vi "Rohde & Schwarz VNA Set Trace Display.vi"(4 "Trace":i8=1 min=1 max=99 step=1, 6 "Channel":i8=1 min=1 max=99 step=1, 7 "Rohde & Schwarz VNA":T1, 8 "error in (no error)":errorcluster, 11 "VISA Resource Name":refnum<visa-resource-name>) -> (0 "error out":errorcluster, 3 "dup VISA Resource Name":refnum<visa-resource-name>)   [LabVIEW 2011]
uses:
  TypeDefs/Rohde & Schwarz VNA Instrument Info.ctl
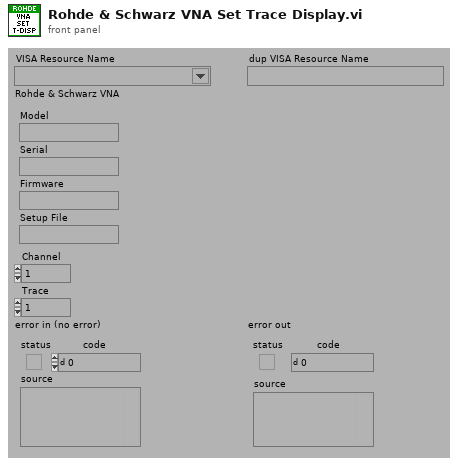
[diagram p1: front panel]
types:
  T1 = typedef "Rohde & Schwarz VNA Instrument Info.ctl" = cluster{"Model":string, "Serial":string, "Firmware":string, "Setup File":string}
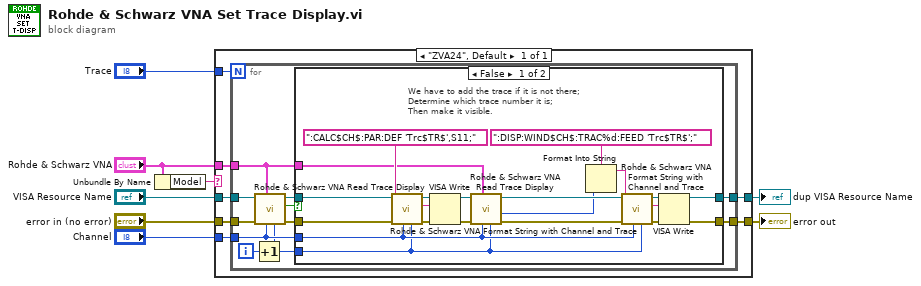
[diagram p0: block diagram]
diagram:
  n1 = Unbundle By Name("Rohde & Schwarz VNA") -> ("Model"=w1:string)
  n2 = case shown="\"ZVA24\", Default" w1 {
    tunnel: "VISA Resource Name" -> [w12]
    tunnel: "error in (no error)" -> [w13]
    tunnel: [w15] -> w6
    tunnel: [w14] -> w5
    tunnel: "Channel" -> [w10]
    tunnel: "Rohde & Schwarz VNA" -> [w11]
    tunnel: "Trace" -> [w9]
    frame "ZVA24", Default {
      n3 = for {
        N: w9 -> [_]
        tunnel: [w26] -> w15
        tunnel: [w25] -> w14
        tunnel: w13 -> [w24]
        tunnel: w12 -> [w23]
        tunnel: w11 -> [w18]
        tunnel: w10 -> [w17]
        i -> [w19]
        n4 = Increment(x=w19) -> (x+1=w16:i32)
        n5 = call "Rohde & Schwarz VNA Read Trace Display.vi"("Trace"=w16, "Channel"=w17, "Rohde & Schwarz VNA"=w18, "error in (no error)"=w24, "VISA Resource Name"=w23) -> ("error out"=w21:errorcluster, "Displayed?"=w20:bool, "dup VISA Resource Name"=w22:refnum<visa-resource-name>)  [unwired: 4 out]
        n6 = case shown="False" w20 {
          tunnel: [w36 w45] -> w26
          tunnel: [w35 w44] -> w25
          tunnel: w22 -> [w43 w45]
          tunnel: w21 -> [w42 w44]
          tunnel: w18 -> [w30 _]
          tunnel: w17 -> [w28 _]
          tunnel: w16 -> [w27 _]
          frame False {
            # "We have to add the trace if it is not there;\nDetermine which trace number it is;\nThen make it visible."
            n7 = call "Rohde & Schwarz VNA Format String with Channel and Trace.vi"("Trace"=w27, "Channel"=w28, "String"=":CALC$CH$:PAR:DEF 'Trc$TR$',S11;" ("write buffer")) -> ("String Out"=w41:string)  [unwired: 6 out]
            n8 = VISA Write(VISA resource name=w43, write buffer=w41, error in (no error)=w42) -> (VISA resource name out=w34:refnum<visa-resource-name>, error out=w33:errorcluster)  [unwired: 1 out]
            n9 = call "Rohde & Schwarz VNA Read Trace Display.vi"("Trace"=w27, "Channel"=w28, "Rohde & Schwarz VNA"=w30, "error in (no error)"=w33, "VISA Resource Name"=w34) -> ("error out"=w32:errorcluster, "Trace Index"=w29:i32, "dup VISA Resource Name"=w31:refnum<visa-resource-name>)  [unwired: 4 out]
            n10 = Format Into String(format string=":DISP:WIND$CH$:TRAC%d:FEED 'Trc$TR$';" ("write buffer"), w29) -> (resulting string=w38:string)  [unwired: 2 in, 1 out]
            n11 = call "Rohde & Schwarz VNA Format String with Channel and Trace.vi"("Trace"=w27, "Channel"=w28, "String"=w38) -> ("String Out"=w37:string)  [unwired: 6 out]
            n12 = VISA Write(VISA resource name=w31, write buffer=w37, error in (no error)=w32) -> (VISA resource name out=w36:refnum<visa-resource-name>, error out=w35:errorcluster)  [unwired: 1 out]
          }
          frame True {
          }
        }
      }
    }
  }
  "dup VISA Resource Name" <- w6
  "error out" <- w5
